vi "integrator.vi"() -> ()   [LabVIEW 2022 SP3]
panel:
  in  "No. cycles":u32
  out "Waveform Graph":dynamicdata(graph)
  in  "Bleed":dbl
  in  "Wait time":u32
  in  "stop":bool
  in  "Noise Ampl":dbl(knob) scale=0.0..1.0
  in  "Frequency":dbl(knob) scale=0.0..10.0
  out "Meter":dbl(knob) scale=-1.0..1.0
  in  "Avg #pts":dbl
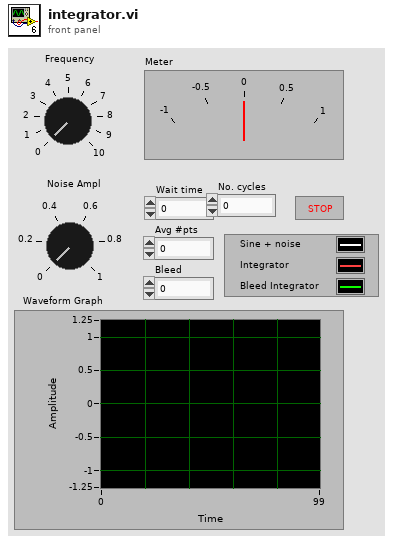
[diagram p1: front panel]
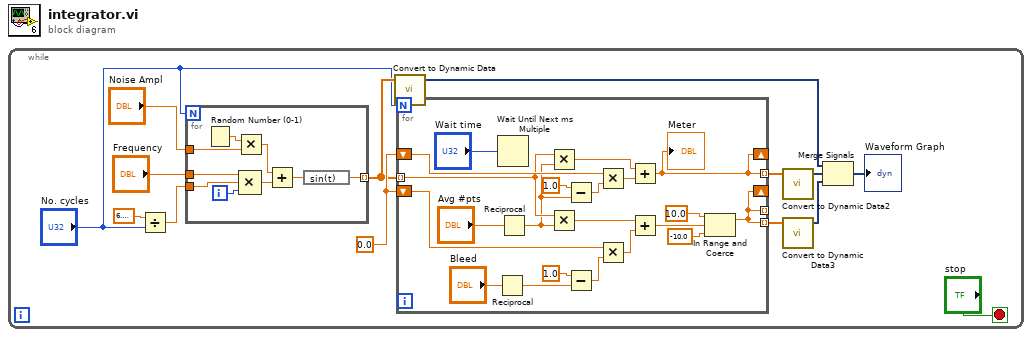
[diagram p0: block diagram]
diagram:
  n1 = while {
    stop <- "stop" stop-if-true
    w9 = 0.0 ("x")
    n2 = Divide(x=6.283185307179586, y="No. cycles") -> (x/y=w11:dbl)
    n3 = for {
      N: "No. cycles" -> [_]
      tunnel: "Noise Ampl" -> [w43]
      tunnel: "Frequency" -> [w41]
      tunnel: [w37] -> w8 mode=indexing
      tunnel: w11 -> [w36]
      i -> [w44]
      n4 = Random Number (0-1)() -> (number: 0 to 1=w42:dbl)
      n5 = Multiply(x=w42, y=w43) -> (x*y=w40:dbl)
      n6 = Compound Arithmetic op=MULTIPLY(w41, w36, w44) -> (w39:dbl)
      n7 = Add(x=w40, y=w39) -> (x+y=w38:dbl)
      n8 = expression code="sin(t)"(w38) -> (w37:dbl)
    }
    n9 = call "Convert to Dynamic Data"("Array"=w8) -> ("Dynamic Data Type"=w7:dynamicdata)  [unwired: 3 in]
    n10 = for {
      N: "No. cycles" -> [_]
      shift-right: [w29] -> _
      shift-left: w9 -> [w33]
      tunnel: [w29] -> w6 mode=indexing
      tunnel: w8 -> [w27] mode=indexing
      shift-right: [w15] -> _
      shift-left: w9 -> [w22]
      tunnel: [w15] -> _ mode=indexing
      tunnel: [w15] -> w4 mode=indexing
      n11 = Reciprocal(x="Bleed") -> (1/x=w23:dbl)
      n12 = Wait Until Next ms Multiple(millisecond multiple="Wait time") -> ()  [unwired: 1 out]
      n13 = Reciprocal(x="Avg #pts") -> (1/x=w26:dbl)
      n14 = Multiply(x=w27, y=w26) -> (x*y=w31:dbl)
      n15 = Multiply(x=w27, y=w26) -> (x*y=w20:dbl)
      n16 = Subtract(x=1.0, y=w26) -> (x-y=w32:dbl)
      n17 = Subtract(x=1.0, y=w23) -> (x-y=w21:dbl)
      n18 = Multiply(x=w33, y=w32) -> (x*y=w30:dbl)
      n19 = Multiply(x=w22, y=w21) -> (x*y=w19:dbl)
      n20 = Add(x=w31, y=w30) -> (x+y=w29:dbl)
      "Meter" <- w29
      n21 = Add(x=w20, y=w19) -> (x+y=w16:dbl)
      n22 = In Range and Coerce(upper limit=10.0 ("x"), x=w16, lower limit=-10.0 ("x")) -> (coerced(x)=w15:dbl)  [unwired: 1 out]
    }
    n23 = call "Convert to Dynamic Data2"("Array"=w6) -> ("Dynamic Data Type"=w5:dynamicdata)  [unwired: 3 in]
    n24 = call "Convert to Dynamic Data3"("Array"=w4) -> ("Dynamic Data Type"=w3:dynamicdata)  [unwired: 3 in]
    n25 = Merge Signals(w7, w5, w3) -> (→"Waveform Graph":dynamicdata)
  }
